vi "Square Wave Generator (Host).vi"() -> ()   [LabVIEW 2012]
doc: "This VI sets the frequency, phase offset, duty cycle, offset, and amplitude for each of three square waves generated on the FPGA."
uses:
  <vilib>/FPGAPlugInAG/PCIe-7841R/niLvFpga_Open_PCIe-7841R.vi
  <vilib>/rvi/interface/common/dynamic/niFpgaDynamicAddResources.vi
  <vilib>/Utility/error.llb/Error Cluster From Error Code.vi
  <vilib>/rvi/errors/niLvFpgaAdjustHostInterfaceError.vi
  <vilib>/FPGAPlugInAG/Dynamic/niLvFpga_Close_Dynamic.vi
  <vilib>/rvi/interface/nirviOpenFPGA/nirviOpenFPGA.xnode
  FPGA Bitfiles/OpticsTable_FPGATarget_SquareWaveGenera_LRUiBB9mKwM.lvbitx
  Square Wave Generator (FPGA).vi
  <vilib>/rvi/interface/nirviReadWriteControl/nirviReadWriteControl.xnode
  <vilib>/rvi/interface/nirviCloseFPGA/nirviCloseFPGA.xnode
  NiFpgaLv.dll
  <vilib>/rvi/interface/Simulation/niFpgaSimulationCallBeginRW.vi
panel:
  in  "Max voltage for target":dbl=10.0
  in  "Clock rate":dbl=40000000.0 format="%#_4p Hz"
  in  "Square wave":T1={"Frequency"=10000.0, "Phase offset"=0.0, "Amplitude (V peak)"=10.0, "Offset (V)"=0.0, "Duty cycle"=50.0} {"Duty cycle" scale=5.0..95.0; "Frequency" format="%#_5p Hz"; "Phase offset" format="%#.2f deg"}
  in  "stop":bool
  in  "Reset":bool
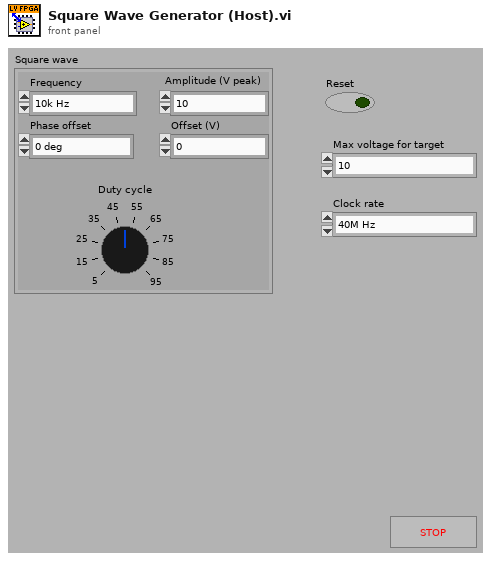
[diagram p1: front panel]
types:
  T1 = cluster{"Frequency":dbl, "Phase offset":dbl, "Amplitude (V peak)":dbl, "Offset (V)":dbl, "Duty cycle":dbl}
  T2 = cluster{"frequency (periods/tick)":fxp<+,32,0>, "phase offset (periods)":fxp<+,32,0>, "amplitude":i16, "offset":i16, "duty cycle (periods)":fxp<+,32,0>}
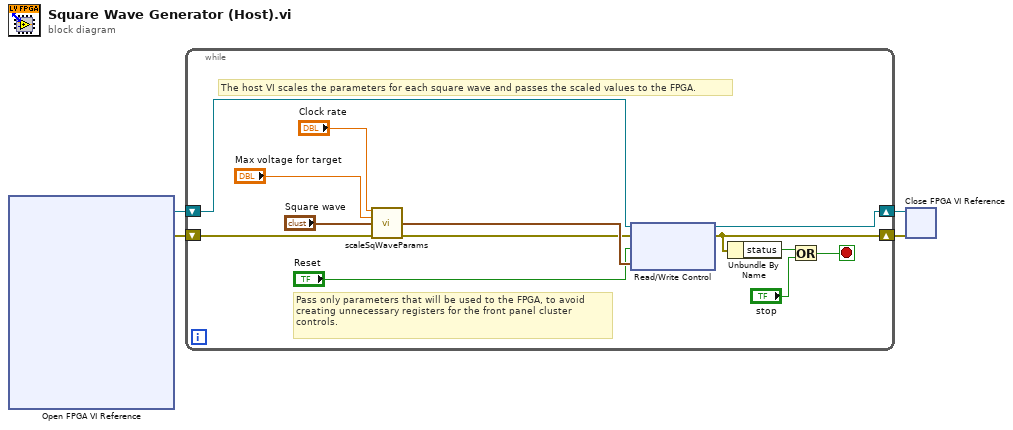
[diagram p0: block diagram]
diagram:
  n1 = xnode "Open FPGA VI Reference"() -> ("FPGA VI Reference Out"=w2:refnum<k20>, "error out"=w1:errorcluster)  [unwired: 2 in]
  n2 = while {
    shift-right: [w10] -> w4
    shift-left: w1 -> [w11]
    shift-right: [w16] -> w3
    shift-left: w2 -> [w17]
    stop <- w7 stop-if-true
    # "Pass only parameters that will be used to the FPGA, to avoid\ncreating unnecessary registers for the front panel cluster\ncontrols."
    # "The host VI scales the parameters for each square wave and passes the scaled values to the FPGA."
    n3 = call "scaleSqWaveParams.vi"("clock rate (Hz)"="Clock rate", "max voltage for target"="Max voltage for target", "square wave props"="Square wave", "error in (no error)"=w11) -> ("scaled square wave props"=w15:T2, "error out"=w5:errorcluster)  [unwired: 10 in]
    n4 = xnode "Read/Write Control"("FPGA VI Reference In"=w17, "error in"=w5, "reset"="Reset", "Square wave"=w15) -> ("FPGA VI Reference Out"=w16:refnum<k20>, "error out"=w10:errorcluster)
    n5 = Unbundle By Name(w10) -> ("status"=w8:bool)
    n6 = Or(x=w8, y="stop") -> (x .or. y?=w7:bool)
  }
  n7 = xnode "Close FPGA VI Reference"("FPGA VI Reference In"=w3, "error in"=w4) -> ()  [unwired: 1 out]
